vi "test.vi"() -> ()   [LabVIEW 2020]
uses:
  <vilib>/Analysis/1siggen.llb/Ramp Pattern by Delta.vi
  <vilib>/Analysis/NI_AALBase.lvlib
panel:
  out "XY Graph":cluster{"X":dbl, "Y":dbl}[](graph)
  out "Labelled Integrals":T1(array[cluster])
  in  "Output File":path=path "Z:/out.txt"
  out "integrals required":i32
  out "Plan in":string
  out "GCode for GRBL":string
  in  "Input File":path=path "Z:/plan.txt"
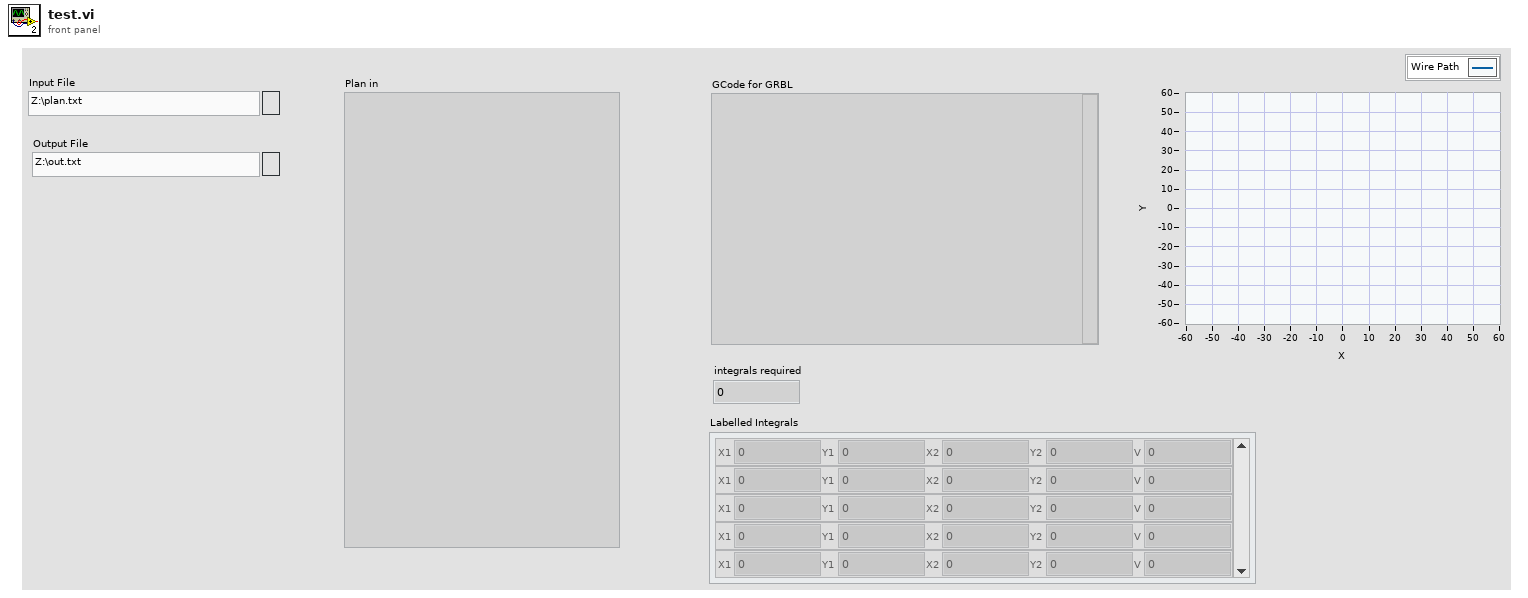
[diagram p1: front panel]
types:
  T1 = cluster{"X1":dbl, "Y1":dbl, "X2":dbl, "Y2":dbl, "V":dbl}[]
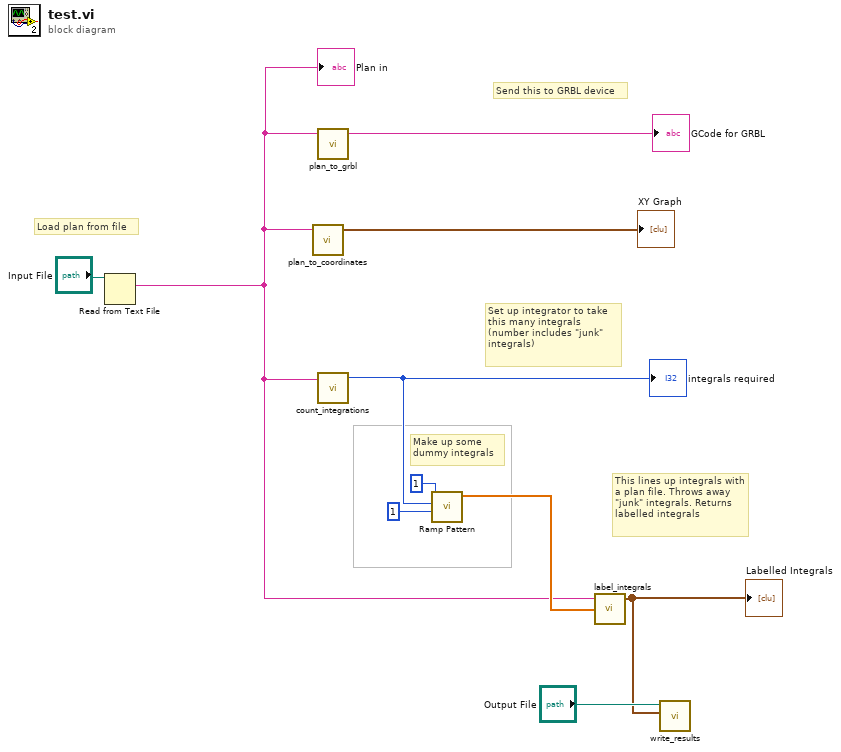
[diagram p0: block diagram]
diagram:
  # "This lines up integrals with a plan file. Throws away \"junk\" integrals. Returns labelled integrals"
  # "Set up integrator to take this many integrals (number includes \"junk\" integrals)"
  # "Send this to GRBL device"
  # "Load plan from file"
  # "Make up some\ndummy integrals"
  n1 = Read from Text File(file (use dialog)="Input File") -> (text=w2:string)  [unwired: 3 in, 3 out]
  "Plan in" <- w2
  n2 = call "plan_to_coordinates.vi"("Plan GCode"=w2) -> ("XY Graph"=→"XY Graph":cluster{"X":dbl, "Y":dbl}[])  [unwired: 3 in, 1 out]
  n3 = call "plan_to_grbl.vi"("Plan GCode"=w2) -> ("GCode for GRBL"=→"GCode for GRBL":string)  [unwired: 3 in, 1 out]
  n4 = call "count_integrations.vi"("Plan"=w2) -> ("integrals required"=w6:i32)  [unwired: 3 in, 1 out]
  "integrals required" <- w6
  n5 = call-poly <vilib>:"Ramp Pattern.vi"("start"=1, "end"=w6, "delta"=1) -> ("Ramp Pattern"=w5:dbl[])  [unwired: 6 in, 2 out]
  n6 = call "label_integrals.vi"("Integrals"=w5, "Plan"=w2) -> ("Labelled Integrals"=w3:T1)  [unwired: 2 in, 1 out]
  "Labelled Integrals" <- w3
  n7 = call "write_results.vi"("Labelled Integrals"=w3, "file path"="Output File") -> ()  [unwired: 9 in, 1 out]
